vi "MainProgram.vi"() -> ()   [LabVIEW 2013]
uses:
  MainProgram/Control/SystemTab.ctl
  MainProgram/Control/StatusInformation.ctl
  MainProgram/Control/Port.ctl
  MainProgram/Control/SystemProcess.ctl
  MainProgram/Control/Read&Write.ctl
  MainProgram/Control/Buffer.vi
panel:
  out "new?":bool
  out "TestBar":i32(slide)=43 min=0 max=75 step=1 scale=0.0..11.0
  out "Information":T1={"PASS:"="", "Barcode(S/N):"="DSF", "TestStep:"=" 43", "TestTime:"="9.44S", "FAIL:"="", "Model:"="91811201R1F-FCT1", "IntervalT:"="", "Status:"="Wait...", "Yield:"="", "Reserve:"="457527"}
  in  "Button-Exit":bool
  in  "Button-Stop":bool
  in  "Button-Test":bool
  out "Result":string="FAIL"
  in  "System-Tab":T2
  in  "TesterBoxs":i32[](listbox)=[6] caption="Prog Boxs:"
  in  "SAVE":bool
  in  "Port":T3={"Multimeter"="USB0::0x2A8D::0x1301::MY53213994::INSTR", "ACsource "="COM12", "GEA"="COM1", "WT200"="COM15", "AutoScan"="COM10", "lines"="Dev0/port0/line0:7, Dev0/port1/line0:7, Dev0/port2/line0:7, Dev0/port3/line0:7, Dev0/port4/line0:7, Dev0/port5/line0:7, Dev0/port6/line0:7, Dev0/port7/line0:7, Dev0/port8/line0:7, Dev0/port9/line0:7, Dev0/port10/line0:7, Dev0/port11/line0:7", "MabeCOM"="COM2"}
  # "Quanta HiPot Tester"
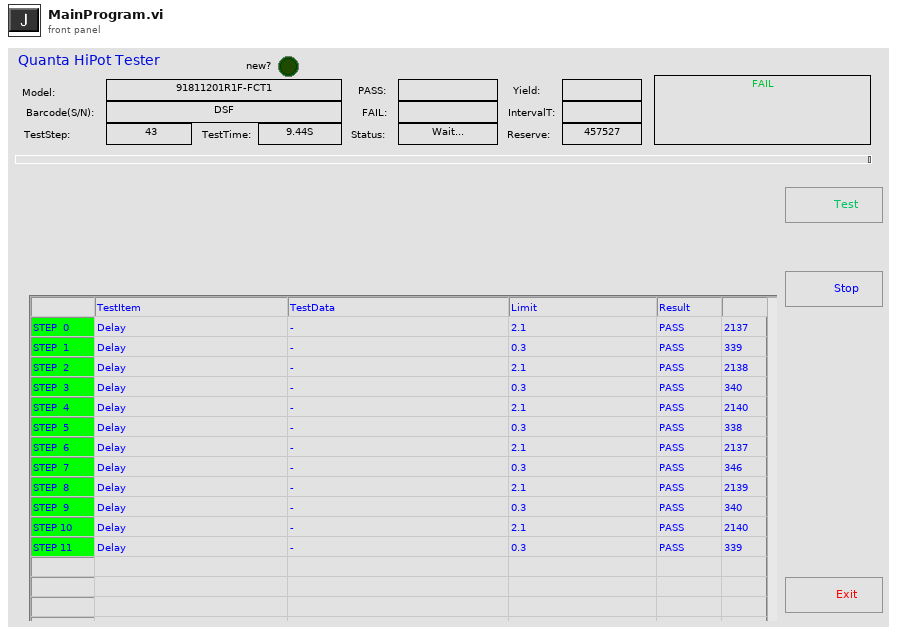
[diagram p1: front panel]
types:
  T1 = typedef "StatusInformation.ctl" = cluster{"PASS:":string, "Barcode(S/N):":string, "TestStep:":string, "TestTime:":string, "FAIL:":string, "Model:":string, "IntervalT:":string, "Status:":string, "Yield:":string, "Reserve:":string}
  T2 = typedef "SystemTab.ctl" = enum32{"Tester", "Set", "Reserve"}
  T3 = typedef "Port.ctl" = cluster{"Multimeter":refnum<visa-resource-name>, "ACsource ":refnum<visa-resource-name>, "GEA":refnum<visa-resource-name>, "WT200":refnum<visa-resource-name>, "AutoScan":refnum<visa-resource-name>, "lines":tag, "MabeCOM":refnum<visa-resource-name>}
  T4 = enum8{"Enabled", "Disabled", "Disabled and Grayed Out"}
  T5 = typedef "SystemProcess.ctl" = enum16{"Idle", "SystemInit", "SpecialEvent", "Barcode(SN)", "TestInitialize", "Test", "Stop", "SaveTestData", "Exit"}
  T6 = cluster{"menu reference":refnum<k9>, "TesterBoxs":refnum<vi>, "TestBar":refnum<vi>, "Information":refnum<vi>, "Result":refnum<vi>, "System-Tab":refnum<vi>, "Port":refnum<vi>}
  T7 = cluster{"pass acess":string[], "fail acess":string, "bad":i32, "time stamp":timestamp, "millisecond timer value":u32}
  T8 = typedef "Read&Write.ctl" = enum16{"Read", "Write"}
  T9 = typedef "TestItemBox.ctl" = cluster{"T/F":bool, "TestItem":T10, "Limit":string, "Describe":string}
  T10 = typedef "TestItem.ctl" = enum16{"Dynamic_call", "idle", "Dialog", "Check_SF", "Delay", "Reset_HiPot", "HV_Test", "GB_Test", "Instrument_Write&Read_HIPOT", "Hipot_ReadResult", "Hipot_Close", "CheckModel", "ScanTestStart", "ScanMultChannel_DCV", "ScanOneChannel_DCV", "Diplay_TestList"}
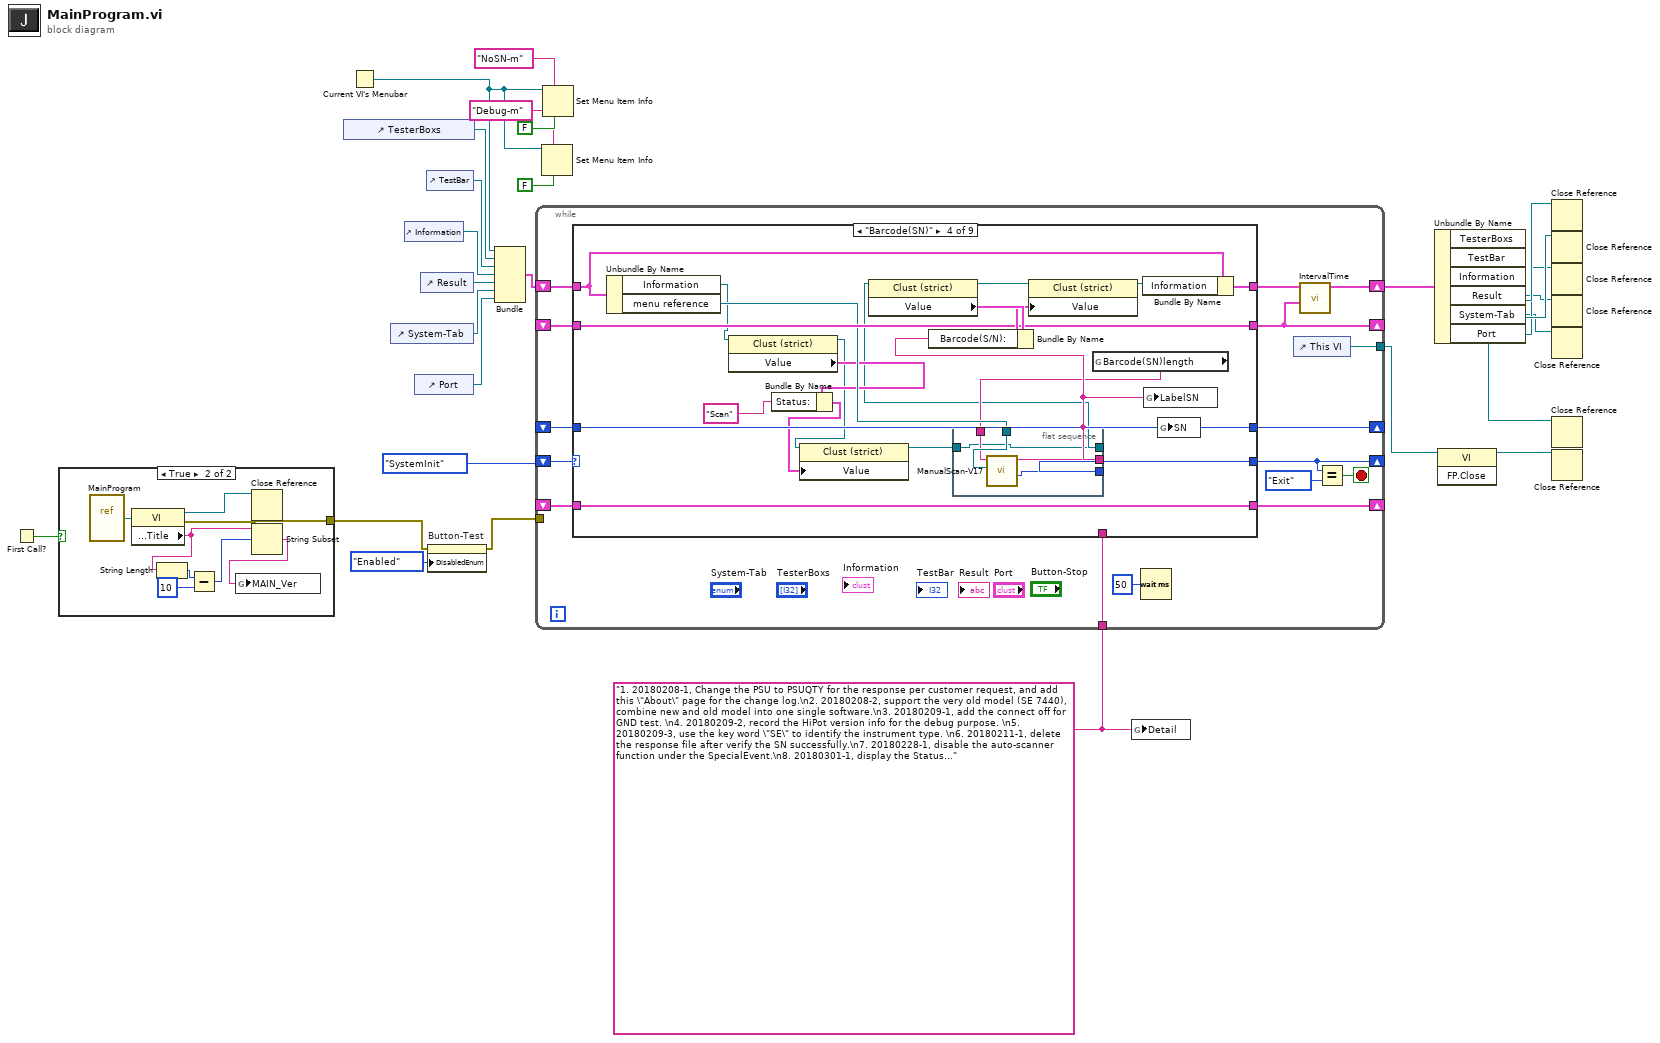
[diagram p0: block diagram]
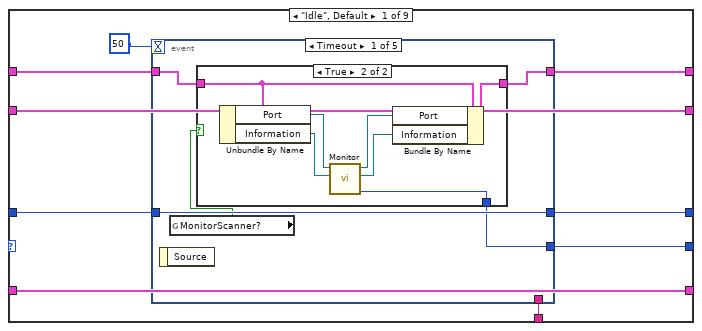
[diagram p3: hidden frame]
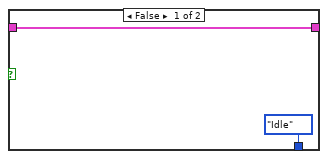
[diagram p4: hidden frame]
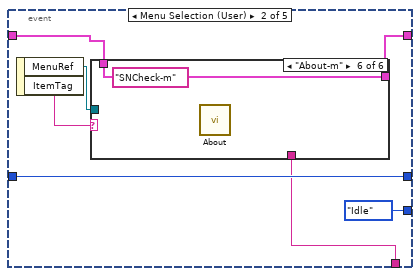
[diagram p5: hidden frame]
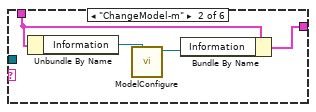
[diagram p7: hidden frame]
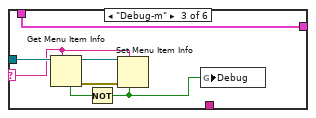
[diagram p8: hidden frame]
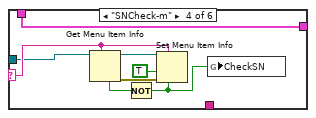
[diagram p9: hidden frame]
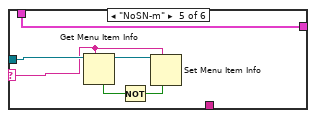
[diagram p10: hidden frame]
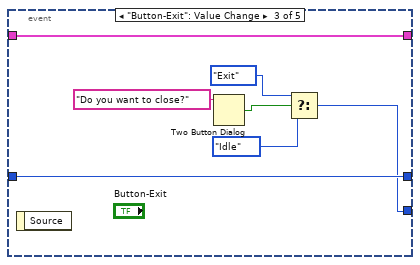
[diagram p11: hidden frame]
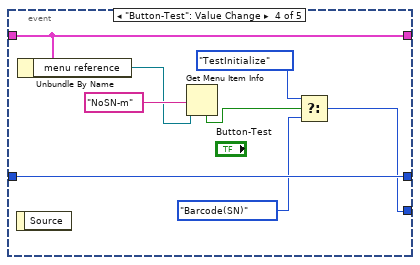
[diagram p12: hidden frame]
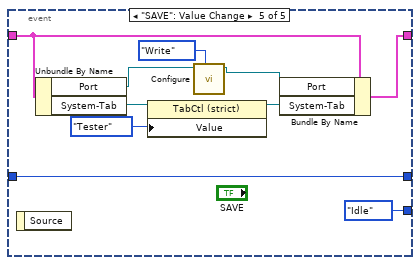
[diagram p13: hidden frame]
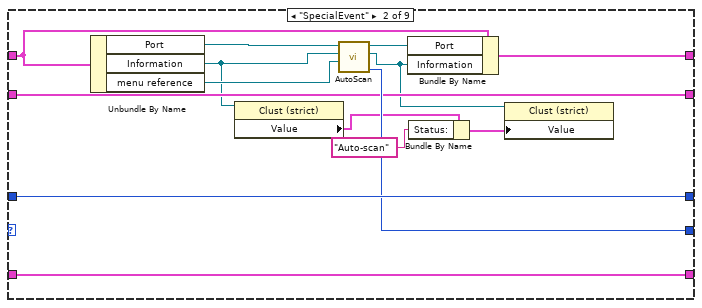
[diagram p14: hidden frame]
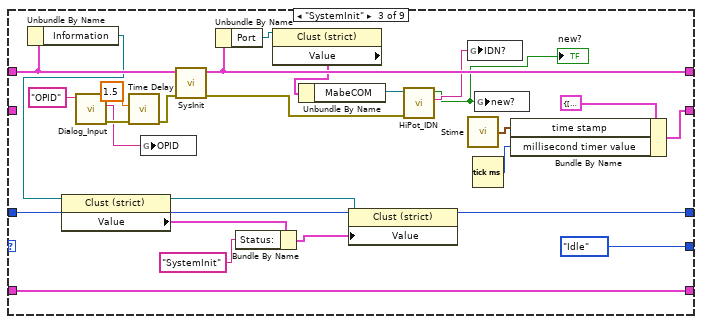
[diagram p15: hidden frame]
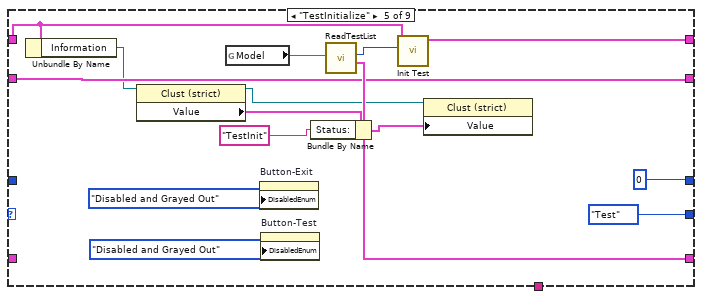
[diagram p16: hidden frame]
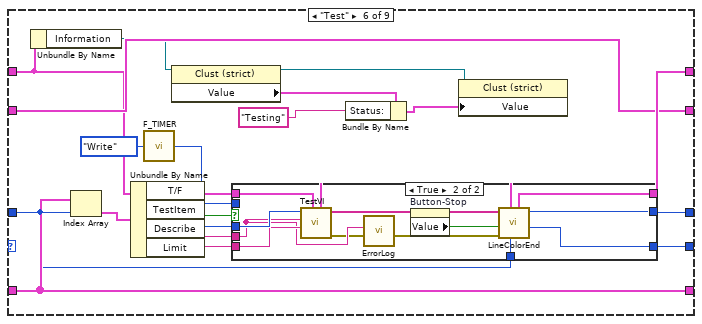
[diagram p17: hidden frame]
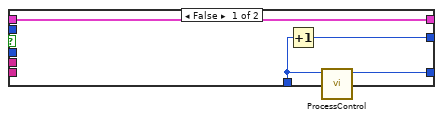
[diagram p18: hidden frame]
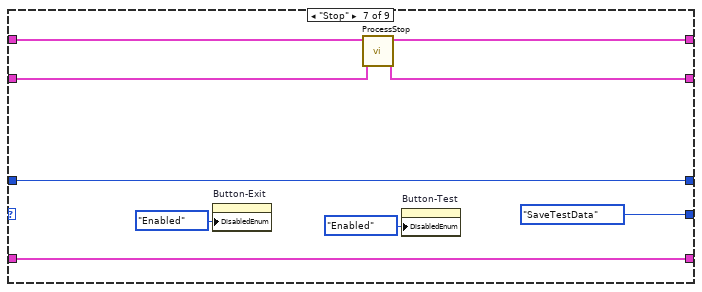
[diagram p19: hidden frame]
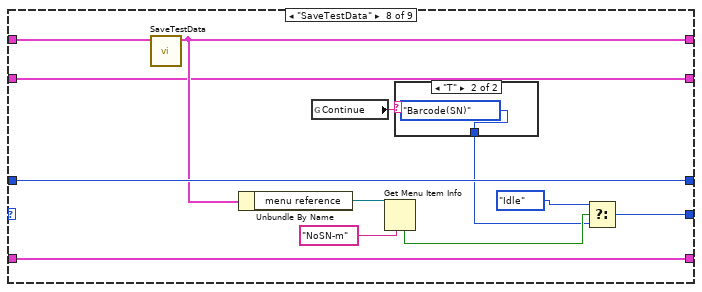
[diagram p20: hidden frame]
diagram:
  w1 = "1. 20180208-1, Change the PSU to PSUQTY for the response per customer request, and add this \"About\" page for the change log.\n2. 20180208-2, support the very old model (SE 7440), combine new and old model into one single software.\n3. 20180209-1, add the connect off for GND test. \n4. 20180209-2, record the HiPot version info for the debug purpose. \n5. 20180209-3, use the key word \"SE\" to identify the instrument type. \n6. 20180211-1, delete the response file after verify the SN successfully.\n7. 20180228-1, disable the auto-scanner function under the SpecialEvent.\n8. 20180301-1, display the Status info for the debug purpose.\n9. 20180302-1, change the hotkey of \"OK\" to END in ManualScan.vi, and filter the string from scanner.\n10. 20180302-2, modify the ManualScan.vi with the \"0D0A\" identification.\n11. 20190313-1, modify the GB_Test.vi with the offset option.\n12. 20190316-1, fix a bug for the GB_Test.vi for the offset function.\n13. 20190318-1, modify the ManualScan-V17.vi with the \"Return\" identification.\n14. 20190328-2, delete the space after the command \"scan\" (both HV_Test.vi and GB_Test.vi) for SE 7440 series."
  n1 = First Call?() -> (First Call?: T/F=w8:bool)
  n2 = case shown="True" w8 {
    tunnel: [_ w34] -> w7
    frame False {
    }
    frame True {
      n3 = vi-ref "MainProgram.vi"() -> (w35:refnum<vi>)
      n4 = property class="VI"(reference=w35) -> (reference out=w33:refnum<vi>, error out=w34:errorcluster, "Front Panel.Title"=w31:string)  [unwired: 1 in]
      n5 = String Length(string=w31) -> (length=w30:i32)
      n6 = Subtract(x=w30, y=10) -> (x-y=w28:i32)
      n7 = Close Reference(reference=w33) -> ()  [unwired: 1 in, 1 out]
      n8 = String Subset(string=w31, offset (0)=w28) -> (substring=w32:string)  [unwired: 1 in]
      n9 = global write "Buffer.vi" "MAIN_Ver"(w32) -> ()
    }
  }
  n10 = control-ref of="TesterBoxs"() -> (w25:refnum<vi>)
  n11 = Current VI's Menubar() -> (w4:refnum<k9>)
  n12 = control-ref of="System-Tab"() -> (w15:refnum<vi>)
  n13 = control-ref of="Information"() -> (w21:refnum<vi>)
  n14 = control-ref of="Port"() -> (w10:refnum<vi>)
  n15 = control-ref of="Result"() -> (w20:refnum<vi>)
  n16 = control-ref of="TestBar"() -> (w26:refnum<vi>)
  n17 = property on="Button-Test" class="Bool"(error in=w7, "DisabledEnum"=T4."Enabled" ("Disabled")) -> (error out=w12:errorcluster)  [unwired: 1 in, 1 out]
  n18 = Bundle("menu reference"=w4, "TesterBoxs"=w25, "TestBar"=w26, "Information"=w21, "Result"=w20, "System-Tab"=w15, "Port"=w10) -> (w9:T6)  [unwired: 1 in]
  n19 = while {
    shift-right: [w50] -> _
    shift-left: SystemProcess."SystemInit" ("MainProcess") -> [w51]
    shift-right: [w38] -> w24
    shift-left: w9 -> [w48]
    tunnel: [w47] -> w17
    shift-right: [w46] -> _
    shift-left: _ -> [w45]
    shift-right: [w43] -> _
    shift-left: _ -> [w44]
    tunnel: w12 -> [_]
    shift-right: [w37] -> _
    shift-left: _ -> [w40]
    tunnel: w1 -> [w36]
    stop <- w41 stop-if-true
    n20 = case shown="\"Barcode(SN)\"" w51 {
      tunnel: [w60 w144 SystemProcess."Idle" ("MainProcess") w192 SystemProcess."Test" ("MainProcess") w227 SystemProcess."SaveTestData" ("MainProcess") w262 SystemProcess."Exit" ("MainProcess")] -> w50
      tunnel: w48 -> [w59 w139 w152 w185 w199 w214 w254 w267 w275]
      tunnel: [w58 w145 w159 w184 w212 w224 w251 w261 w275] -> w39
      tunnel: [w57 w147 w171 w191 w208 w231 w256 w269 w274] -> w46
      tunnel: w45 -> [w57 w147 w171 w191 _ w231 w256 w269 w274]
      tunnel: w44 -> [w54 w146 w170 w190 _ w226 w255 w268 w273]
      tunnel: [w55 w146 w170 w190 0 w225 w255 w268 w273] -> w43
      tunnel: w40 -> [w53 w141 _ w182 w206 w219 w250 w260 w272]
      tunnel: [w53 w141 w167 w182 w206 w219 w249 w260 w272] -> w37
      tunnel: w36 -> [w52 _ _ _ _ _ _ _ _]
      frame "Idle", Default {
        n21 = event shown="[0] Timeout" {
          selector: _ -> [_ _ _ _ _]
          dyn-events: _ -> [_ _ _ _ _]
          timeout: 50 -> [_ _ _ _ _]
          tunnel: [w62 SystemProcess."Idle" ("MainProcess") w111 w117 SystemProcess."Idle" ("MainProcess")] -> w60
          tunnel: w59 -> [w64 w79 w114 w122 w129]
          tunnel: [w63 w78 w114 w122 w128] -> w58
          tunnel: [w65 w80 w115 w123 w127] -> w55
          tunnel: w54 -> [w65 w80 w115 w123 w127]
          tunnel: w52 -> [_ w75 _ _ _]
          event Timeout {
            n22 = event-data() -> ()  [unwired: 1 in, 1 out]
            n23 = global read "Buffer.vi" "MonitorScanner?"() -> (w61:bool)
            n24 = case shown="True" w61 {
              tunnel: w64 -> [w66 w74]
              tunnel: [w66 w73] -> w63
              tunnel: [SystemProcess."Idle" ("Process") w72] -> w62
              frame False {
              }
              frame True {
                n25 = Unbundle By Name(w74) -> ("Port"=w69:refnum<vi>, "Information"=w71:refnum<vi>)
                n26 = call "Monitor.vi"("Information"=w71, "Port 2"=w69) -> ("Process"=w72:T5, "Information"=w70:refnum<vi>, "reference out"=w68:refnum<vi>)  [unwired: 7 in]
                n27 = Bundle By Name(cluster=w74, "Port"=w68, "Information"=w70) -> (w73:T6)
              }
            }
          }
          event Menu Selection (User) {
            (unwired) "SNCheck-m" ("ItemTag")
            n28 = event-data() -> ("MenuRef"=w77:refnum<k9>, "ItemTag"=w76:string)  [unwired: 1 in]
            n29 = case shown="\"About-m\"" w76 {
              selector: w76 -> [_ _ w91 w99 w103 _]
              tunnel: [w82 w86 w88 w96 w102 w108] -> w78
              tunnel: w77 -> [_ _ w93 w97 w104 _]
              tunnel: w79 -> [w82 w83 w88 w96 w102 w108]
              tunnel: w75 -> [_ _ _ _ _ _]
              frame Default {
              }
              frame "ChangeModel-m" {
                n30 = Unbundle By Name(w83) -> ("Information"=w85:refnum<vi>)
                n31 = call "ModelConfigure.vi"("Cluster in"=w85) -> ("Cluster out"=w84:refnum<vi>)  [unwired: 10 in]
                n32 = Bundle By Name(cluster=w83, "Information"=w84) -> (w86:T6)
              }
              frame "Debug-m" {
                n33 = Get Menu Item Info(7:w91, 11:w93) -> (0:w89:errorcluster, 3:w92:refnum<k9>, 4:w90:bool)  [unwired: 1 in, 4 out]
                n34 = Not(x=w90) -> (.not. x?=w87:bool)
                n35 = Set Menu Item Info(6:w87, 7:w91, 8:w89, 11:w92) -> ()  [unwired: 3 in, 2 out]
                n36 = global write "Buffer.vi" "Debug"(w87) -> ()
              }
              frame "SNCheck-m" {
                n37 = Get Menu Item Info(7:w99, 11:w97) -> (0:w98:errorcluster, 3:w101:refnum<k9>, 4:w100:bool)  [unwired: 1 in, 4 out]
                n38 = Not(x=w100) -> (.not. x?=w94:bool)
                n39 = Set Menu Item Info(6:w94, 7:w99, 8:w98, 9:TRUE ("enabled"), 11:w101) -> ()  [unwired: 2 in, 2 out]
                n40 = global write "Buffer.vi" "CheckSN"(w94) -> ()
              }
              frame "NoSN-m" {
                n41 = Get Menu Item Info(7:w103, 11:w104) -> (3:w107:refnum<k9>, 4:w106:bool)  [unwired: 1 in, 5 out]
                n42 = Not(x=w106) -> (.not. x?=w105:bool)
                n43 = Set Menu Item Info(6:w105, 7:w103, 11:w107) -> ()  [unwired: 4 in, 2 out]
              }
              frame "About-m" {
                n44 = call "About.vi"() -> ()  [unwired: 12 in]
              }
            }
          }
          event "Button-Exit": Value Change {
            n45 = event-data() -> ()  [unwired: 1 in, 1 out]
            n46 = Two Button Dialog(message="Do you want to close?") -> (T button?=w113:bool)  [unwired: 2 in]
            n47 = Select(t=SystemProcess."Exit" ("MainProcess"), s=w113, f=SystemProcess."Idle") -> (s? t:f=w111:T5)
          }
          event "Button-Test": Value Change {
            n48 = event-data() -> ()  [unwired: 1 in, 1 out]
            n49 = Unbundle By Name(w122) -> ("menu reference"=w120:refnum<k9>)
            n50 = Get Menu Item Info(7:"NoSN-m" ("item tag"), 11:w120) -> (4:w119:bool)  [unwired: 1 in, 6 out]
            n51 = Select(t=SystemProcess."TestInitialize", s=w119, f=SystemProcess."Barcode(SN)" ("MainProcess")) -> (s? t:f=w117:T5)
          }
          event "SAVE": Value Change {
            n52 = event-data() -> ()  [unwired: 1 in, 1 out]
            n53 = Unbundle By Name(w129) -> ("Port"=w125:refnum<vi>, "System-Tab"=w132:refnum<vi>)
            n54 = property class="TabCtl (strict)"(reference=w132, "Value"=enum32{"Tester", "Set", "Reserve"}."Tester") -> (reference out=w131:refnum<vi>)  [unwired: 1 in, 1 out]
            n55 = call "Configure.vi"("Enum"=enum16{"Read", "Write"}."Write", "Port 4"=w125) -> ("Port 5"=w124:refnum<vi>)  [unwired: 9 in]
            n56 = Bundle By Name(cluster=w129, "Port"=w124, "System-Tab"=w131) -> (w128:T6)
          }
        }
      }
      frame "SpecialEvent" {
        n57 = Unbundle By Name(w139) -> ("Port"=w143:refnum<vi>, "Information"=w137:refnum<vi>, "menu reference"=w140:refnum<k9>)
        n58 = property class="Clust (strict)"(reference=w137) -> ("Value"=w136:T1)  [unwired: 1 in, 2 out]
        n59 = call "AutoScan.vi"("menu reference"=w140, "Information"=w137, "Port 2"=w143) -> ("Process"=w144:T5, "Information"=w138:refnum<vi>, "reference out"=w142:refnum<vi>)  [unwired: 6 in]
        n60 = Bundle By Name(cluster=w139, "Port"=w142, "Information"=w138) -> (w145:T6)
        n61 = Bundle By Name(cluster=w136, "Status:"="Auto-scan") -> (w135:T1)
        n62 = property class="Clust (strict)"(reference=w138, "Value"=w135) -> ()  [unwired: 1 in, 2 out]
      }
      frame "SystemInit" {
        n63 = Unbundle By Name(w152) -> ("Information"=w151:refnum<vi>)
        n64 = property class="Clust (strict)"(reference=w151) -> (reference out=w150:refnum<vi>, "Value"=w149:T1)  [unwired: 1 in, 1 out]
        n65 = call "Dialog_Input.vi"("Caption.Text"="OPID") -> ("error out"=w164:errorcluster, "String out"=w161:string)  [unwired: 8 in, 1 out]
        n66 = call "Time Delay"("error in (no error)"=w164, "Delay Time (s)"=1.5) -> ("error out"=w165:errorcluster)  [unwired: 9 in]
        n67 = global write "Buffer.vi" "OPID"(w161) -> ()
        n68 = call "SysInit.vi"("error in (no error)"=w165, "Cluster"=w152) -> ("error out"=w160:errorcluster, "output cluster"=w159:T6)  [unwired: 8 in]
        n69 = Unbundle By Name(w159) -> ("Port"=w158:refnum<vi>)
        n70 = Bundle By Name(cluster=w149, "Status:"="SystemInit") -> (w148:T1)
        n71 = property class="Clust (strict)"(reference=w158) -> ("Value"=w157:T3)  [unwired: 1 in, 2 out]
        n72 = Unbundle By Name(w157) -> ("MabeCOM"=w156:refnum<visa-resource-name>)
        n73 = property class="Clust (strict)"(reference=w150, "Value"=w148) -> ()  [unwired: 1 in, 2 out]
        n74 = call "HiPot_IDN.vi"("error in (no error)"=w160, "VISA Refnum in"=w156) -> ("read buffer"=w155:string, "new?"=w154:bool)  [unwired: 7 in, 1 out]
        "new?" <- w154
        n75 = global write "Buffer.vi" "IDN?"(w155) -> ()
        n76 = call "Stime.vi"() -> ("time stamp"=w168:timestamp)  [unwired: 2 in, 1 out]
        n77 = Tick Count (ms)() -> (millisecond timer value=w166:u32)
        n78 = global write "Buffer.vi" "new?"(w154) -> ()
        n79 = Bundle By Name(cluster=T7 {"pass acess"=[], "fail acess"="", "bad"=0, "time stamp"=timestamp(0 s since 1904-01-01), "millisecond timer value"=0} ("Cluster"), "time stamp"=w168, "millisecond timer value"=w166) -> (w167:T7)
      }
      frame "Barcode(SN)" {
        n80 = Unbundle By Name(w185) -> ("Information"=w179:refnum<vi>, "menu reference"=w181:refnum<k9>)
        n81 = property class="Clust (strict)"(reference=w179) -> (reference out=w173:refnum<vi>, "Value"=w178:T1)  [unwired: 1 in, 1 out]
        n82 = Bundle By Name(cluster=w178, "Status:"="Scan") -> (w177:T1)
        n83 = property class="Clust (strict)"(reference=w173, "Value"=w177) -> (reference out=w175:refnum<vi>)  [unwired: 1 in, 1 out]
        n84 = property class="Clust (strict)"(reference=w174) -> (reference out=w188:refnum<vi>, "Value"=w189:T1)  [unwired: 1 in, 1 out]
        n85 = Bundle By Name(cluster=w189, "Barcode(S/N):"=w183) -> (w187:T1)
        n86 = flat-sequence {
          tunnel: [w197] -> w192
          tunnel: [w196] -> w183
          tunnel: w181 -> [w195]
          tunnel: w180 -> [w194]
          tunnel: w175 -> [w193]
          tunnel: [w193] -> w174
          frame #0 {
            n87 = call "ManualScan-V17.vi"("menu reference"=w195, "SN Length"=w194) -> ("MainProcess"=w197:T5, "Barcode out:"=w196:string)  [unwired: 8 in]
          }
        }
        n88 = property class="Clust (strict)"(reference=w188, "Value"=w187) -> (reference out=w186:refnum<vi>)  [unwired: 1 in, 1 out]
        n89 = global read "Buffer.vi" "Barcode(SN)length"() -> (w180:string)
        n90 = Bundle By Name(cluster=w185, "Information"=w186) -> (w184:T6)
        n91 = global write "Buffer.vi" "LabelSN"(w183) -> ()
        n92 = global write "Buffer.vi" "SN"(w183) -> ()
      }
      frame "TestInitialize" {
        n93 = Unbundle By Name(w199) -> ("Information"=w198:refnum<vi>)
        n94 = property class="Clust (strict)"(reference=w198) -> (reference out=w202:refnum<vi>, "Value"=w201:T1)  [unwired: 1 in, 1 out]
        n95 = global read "Buffer.vi" "Model"() -> (w204:string)
        n96 = property on="Button-Exit" class="Bool"("DisabledEnum"=T4."Disabled and Grayed Out" ("Disabled")) -> ()  [unwired: 2 in, 2 out]
        n97 = property on="Button-Test" class="Bool"("DisabledEnum"=T4."Disabled and Grayed Out" ("Disabled")) -> ()  [unwired: 2 in, 2 out]
        n98 = Bundle By Name(cluster=w201, "Status:"="TestInit") -> (w200:T1)
        n99 = call "ReadTestList.vi"("Model"=w204) -> ("TestList"=w208:T9[], "size(s)"=w207:i32)  [unwired: 9 in]
        n100 = call "Init Test.vi"("x"=w207, "Cluster"=w199) -> ("output cluster"=w212:T6)  [unwired: 9 in]
        n101 = property class="Clust (strict)"(reference=w202, "Value"=w200) -> ()  [unwired: 1 in, 2 out]
      }
      frame "Test" {
        n102 = Unbundle By Name(w214) -> ("Information"=w213:refnum<vi>)
        n103 = Index Array(array=w231, index=w226) -> (element=w230:T9)
        n104 = Unbundle By Name(w230) -> ("T/F"=w228:bool, "TestItem"=w229:T10, "Describe"=w220:string, "Limit"=w221:string)
        n105 = call "F_TIMER.vi"("Enum-Read/Write"=Read&Write."Write") -> ("timer"=w223:u32)
        n106 = property class="Clust (strict)"(reference=w213) -> (reference out=w217:refnum<vi>, "Value"=w216:T1)  [unwired: 1 in, 1 out]
        n107 = case shown="True" w228 {
          tunnel: w229 -> [_ w248]
          tunnel: w221 -> [_ w244]
          tunnel: [w233 w246] -> w227
          tunnel: w226 -> [w234 w247]
          tunnel: [w235 w245] -> w225
          tunnel: w214 -> [w232 w240]
          tunnel: [w232 w242] -> w224
          tunnel: w223 -> [_ _]
          tunnel: w220 -> [_ w238]
          frame False {
            n108 = Increment(x=w234) -> (x+1=w235:i32)
            n109 = call "ProcessControl.vi"("Row"=w234) -> ("Process"=w233:T5)  [unwired: 10 in]
          }
          frame True {
            n110 = call "TestVI.vi"("Cluster in"=w240, "Limit"=w244, "Describe"=w238, "TestItem"=w248) -> ("Error Out"=w237:errorcluster, "Result\n0.Item\n1.data\n2.limit\n3.result"=w243:string[], "Cluster out"=w239:T6)  [unwired: 5 in]
            n111 = call "ErrorLog.vi"("error in (no error)"=w237, "Step No."=w238) -> ("error out"=w236:errorcluster)  [unwired: 9 in]
            n112 = property on="Button-Stop" class="Bool (strict)"() -> ("Value"=w241:bool)  [unwired: 2 in, 2 out]
            n113 = call "LineColorEnd.vi"("Row"=w247, "Cluster"=w239, "error in"=w236, "Event"=w241, "Result\n0.Item\n1.data\n2.limit\n3.result"=w243) -> ("SystemProcess"=w246:T5, "Row"=w245:i32, "output cluster"=w242:T6)  [unwired: 4 in]
          }
        }
        n114 = Bundle By Name(cluster=w216, "Status:"="Testing") -> (w215:T1)
        n115 = property class="Clust (strict)"(reference=w217, "Value"=w215) -> ()  [unwired: 1 in, 2 out]
      }
      frame "Stop" {
        n116 = property on="Button-Exit" class="Bool"("DisabledEnum"=T4."Enabled" ("Disabled")) -> ()  [unwired: 2 in, 2 out]
        n117 = call "ProcessStop.vi"("Cluster in"=w250, "Cluster"=w254) -> ("Cluster out"=w249:T7, "output cluster"=w251:T6)  [unwired: 8 in]
        n118 = property on="Button-Test" class="Bool"("DisabledEnum"=T4."Enabled" ("Disabled")) -> ()  [unwired: 2 in, 2 out]
      }
      frame "SaveTestData" {
        n119 = call "SaveTestData.vi"("Cluster"=w267) -> ("output cluster"=w261:T6)  [unwired: 9 in, 1 out]
        n120 = Unbundle By Name(w261) -> ("menu reference"=w265:refnum<k9>)
        n121 = global read "Buffer.vi" "Continue"() -> (w259:string)
        n122 = Get Menu Item Info(7:"NoSN-m" ("item tag"), 11:w265) -> (4:w264:bool)  [unwired: 1 in, 6 out]
        n123 = case shown="\"T\"" w259 {
          tunnel: [SystemProcess."Idle" ("MainProcess") SystemProcess."Barcode(SN)" ("MainProcess")] -> w258
          frame Default {
          }
          frame "T" {
          }
        }
        n124 = Select(t=SystemProcess."Idle", s=w264, f=w258) -> (s? t:f=w262:T5)
      }
      frame "Exit" {
      }
    }
    n125 = Wait (ms)(milliseconds to wait=u32 50) -> ()  [unwired: 1 out]
    n126 = control-ref of="This VI"() -> (w47:refnum<vi>)
    n127 = call "IntervalTime.vi"("Cluster out"=w37, "output cluster"=w39) -> ("output cluster 2"=w38:T6)  [unwired: 8 in, 1 out]
    n128 = Equal?(x=w50, y=SystemProcess."Exit" ("MainProcess")) -> (x = y?=w41:bool)
  }
  n129 = Set Menu Item Info(6:FALSE ("checked"), 7:"Debug-m" ("item tag"), 11:w4) -> ()  [unwired: 4 in, 2 out]
  n130 = Set Menu Item Info(6:FALSE, 7:"NoSN-m" ("item tag"), 11:w4) -> ()  [unwired: 4 in, 2 out]
  n131 = global write "Buffer.vi" "Detail"(w1) -> ()
  n132 = Unbundle By Name(w24) -> ("TesterBoxs"=w23:refnum<vi>, "TestBar"=w22:refnum<vi>, "Information"=w19:refnum<vi>, "Result"=w18:refnum<vi>, "System-Tab"=w14:refnum<vi>, "Port"=w13:refnum<vi>)
  n133 = invoke class="VI" method="FP.Close"(reference=w17) -> (reference out=w16:refnum<vi>)  [unwired: 2 in, 2 out]
  n134 = Close Reference(reference=w23) -> ()  [unwired: 1 in, 1 out]
  n135 = Close Reference(reference=w22) -> ()  [unwired: 1 in, 1 out]
  n136 = Close Reference(reference=w19) -> ()  [unwired: 1 in, 1 out]
  n137 = Close Reference(reference=w18) -> ()  [unwired: 1 in, 1 out]
  n138 = Close Reference(reference=w14) -> ()  [unwired: 1 in, 1 out]
  n139 = Close Reference(reference=w13) -> ()  [unwired: 1 in, 1 out]
  n140 = Close Reference(reference=w16) -> ()  [unwired: 1 in, 1 out]
